vi "SetPanelOrigin.vi"(8 "error in (no error)":errorcluster, 11 "VI in":refnum<vi>) -> (0 "error out":errorcluster)   [LabVIEW 2024, in "Application.lvclass"]
uses:
  Application.lvclass
  <vilib>/Utility/miscctls.llb/LVPointTypeDef.ctl
  Application.lvclass/Application.ctl
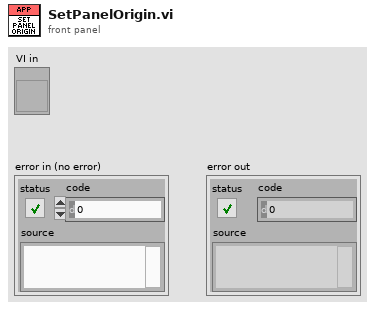
[diagram p1: front panel]
types:
  T1 = typedef "LVPointTypeDef.ctl" = cluster{"Horizontal":i16, "Vertical":i16}
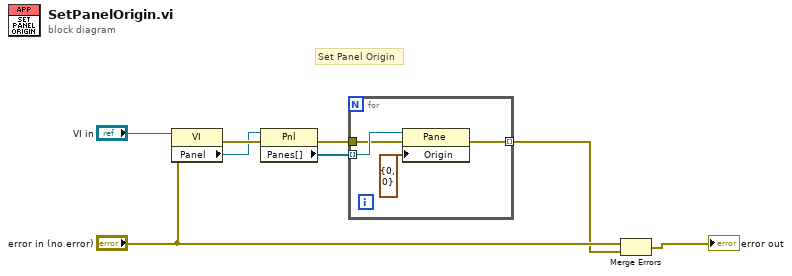
[diagram p0: block diagram]
diagram:
  # "Set Panel Origin"
  n1 = property class="VI"(reference="VI in", error in="error in (no error)") -> (error out=w4:errorcluster, "Panel"=w3:refnum<vi>)  [unwired: 1 out]
  n2 = property class="Pnl"(reference=w3, error in=w4) -> (error out=w6:errorcluster, "Panes[]"=w5:refnum<vi>[])  [unwired: 1 out]
  n3 = for {
    tunnel: w5 -> [w12] mode=indexing
    tunnel: w6 -> [w10]
    tunnel: [w9] -> w1 mode=indexing
    n4 = property class="Pane"(reference=w12, error in=w10, "Origin"=T1 {"Horizontal"=0, "Vertical"=0}) -> (error out=w9:errorcluster)  [unwired: 1 out]
  }
  n5 = Merge Errors("error in (no error)", w1) -> (→"error out":errorcluster)
